vi "Top.vi"() -> ()   [LabVIEW 2020]
uses:
  PowerLineId.ctl
  PowerLineQuantity.ctl
  <vilib>/DAQmx/read.llb/DAQmx Read (Analog 1D Wfm NChan NSamp).vi
  <vilib>/DAQmx/configure/timing.llb/DAQmx Timing (Sample Clock).vi
  <vilib>/DAQmx/configure/task.llb/DAQmx Configure Logging (TDMS).vi
  <extravilib>/ChannelInstances/Messenger-a[.](wfm(dbl))/Instantiate.vi
  <extravilib>/ChannelInstances/Messenger-a[.](wfm(dbl))/Endpoint.vi
  <vilib>/DAQmx/miscellaneous.llb/DAQmx Fill In Error Info.vi
  <extravilib>/ChannelInstances/Messenger-a[.](wfm(dbl)).lvlib
panel:
  in  "Logging Mode":i32(ring)=15842 items=["Off"=10231, "Log"=15844, "Log and Read"=15842]
  in  "Data Read Interval [s]":dbl(knob)=1.0 min=1.0 max=10.0 step=1.0 scale=1.0..10.0 scale format="%#_1f"
  out "Monitor":waveform(dbl)[](graph)
  in  "STOP":bool
  in  "Rate Selection":enum32{"Auto", "Manual"}(radio)
  in  "Sampling Rate [Hz]":dbl(knob)=100000.0 min=100000.0 max=2000000.0 step=50000.0 scale=100000.0..2000000.0 scale format="%.1p"
  in  "Log File Path":path
  in  "START":bool
  in  "Channel\nIO":tag="PXIe-4309/ai2"
  in  "Channel\nPCIEVPH":tag="PXIe-4309/ai5"
  in  "Channel\nDDR_VPP":tag="PXIe-4309/ai15"
  in  "Enable Channel\nIO":bool=TRUE
  in  "Enable Channel\nPCIEVPH":bool=TRUE
  in  "Enable Channel\nDDR_VPP":bool=TRUE
  in  "Channel\nDDR_SOC":tag="PXIe-4309/ai1"
  in  "Channel\nPCIEVP":tag="PXIe-4309/ai4"
  in  "Channel\nDDR_PLL":tag="PXIe-4309/ai7"
  in  "Enable Channel\nDDR_SOC":bool=TRUE
  in  "Enable Channel\nPCIEVP":bool=TRUE
  in  "Enable Channel\nDDR_PLL":bool=TRUE
  in  "Enable Channel\nDDR_MEM":bool=TRUE
  in  "Enable Channel\nPLL":bool=TRUE
  in  "Enable Channel\nCORE":bool=TRUE
  in  "Channel\nDDR_MEM":tag="PXIe-4309/ai6"
  in  "Channel\nPLL":tag="PXIe-4309/ai3"
  in  "Channel\nCORE":tag="PXIe-4309/ai0"
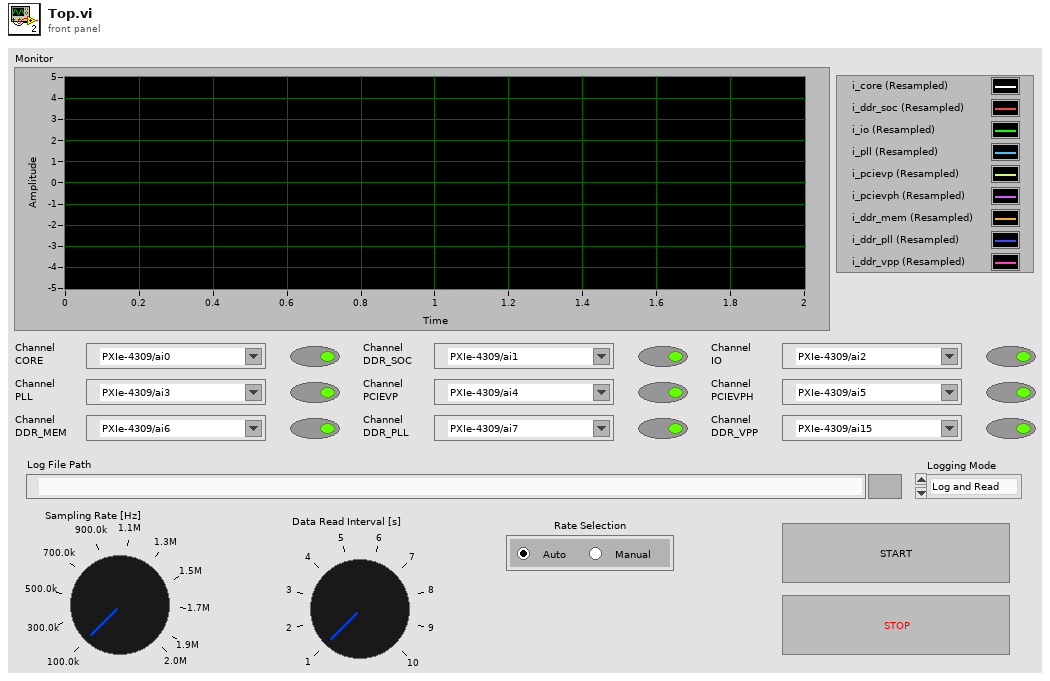
[diagram p1: front panel]
types:
  T1 = typedef "PowerLineId.ctl" = enum8{"CORE", "DDR_SOC", "IO", "PLL", "PCIEVP", "PCIEVPH", "DDR_MEM", "DDR_PLL", "DDR_VPP"}
  T2 = typedef "PowerLineQuantity.ctl" = enum16{"Current", "Voltage"}
  T3 = typedef "PowerLineConfig.ctl" = cluster{"Line Name":string, "Shunt Resistor [Ohm]":dbl, "Min Current [A]":dbl, "Max Current [A]":dbl}
  T4 = typedef "Messenger-a[.](wfm(dbl)).lvlib/))Channel.ctl" = refnum<queue>
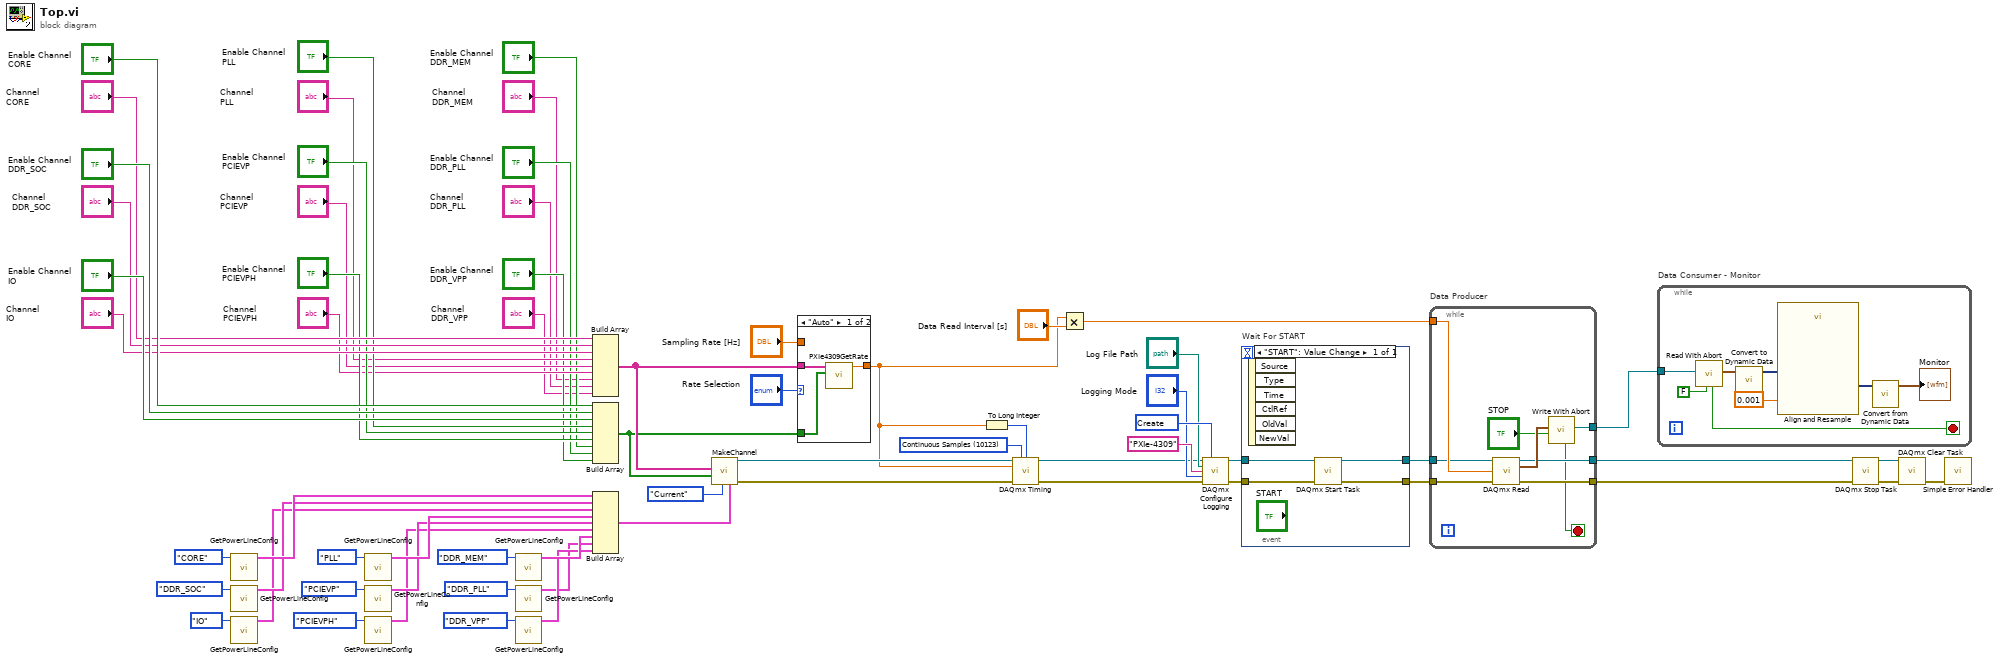
[diagram p0: block diagram]
diagram:
  w33 = 15848 items=["Open"=10437, "Open or Create"=15846, "Create or Replace"=15847, "Create"=15848] ("operation")
  w36 = 10123 items=["Finite Samples"=10178, "Continuous Samples"=10123, "Hardware Timed Single Point"=12522] ("sample mode")
  n1 = call "GetPowerLineConfig.vi"("Power Line\nIdentifier"=PowerLineId."CORE" ("Power Line Identifier")) -> ("Power Line\nConfiguration"=w64:T3)  [unwired: 8 in]
  n2 = call "GetPowerLineConfig.vi"("Power Line\nIdentifier"=PowerLineId."DDR_SOC" ("Power Line Identifier")) -> ("Power Line\nConfiguration"=w63:T3)  [unwired: 8 in]
  n3 = call "GetPowerLineConfig.vi"("Power Line\nIdentifier"=PowerLineId."IO" ("Power Line Identifier")) -> ("Power Line\nConfiguration"=w62:T3)  [unwired: 8 in]
  n4 = call "GetPowerLineConfig.vi"("Power Line\nIdentifier"=PowerLineId."PLL" ("Power Line Identifier")) -> ("Power Line\nConfiguration"=w61:T3)  [unwired: 8 in]
  n5 = call "GetPowerLineConfig.vi"("Power Line\nIdentifier"=PowerLineId."PCIEVP" ("Power Line Identifier")) -> ("Power Line\nConfiguration"=w60:T3)  [unwired: 8 in]
  n6 = call "GetPowerLineConfig.vi"("Power Line\nIdentifier"=PowerLineId."PCIEVPH" ("Power Line Identifier")) -> ("Power Line\nConfiguration"=w59:T3)  [unwired: 8 in]
  n7 = call "GetPowerLineConfig.vi"("Power Line\nIdentifier"=PowerLineId."DDR_MEM" ("Power Line Identifier")) -> ("Power Line\nConfiguration"=w58:T3)  [unwired: 8 in]
  n8 = call "GetPowerLineConfig.vi"("Power Line\nIdentifier"=PowerLineId."DDR_PLL" ("Power Line Identifier")) -> ("Power Line\nConfiguration"=w56:T3)  [unwired: 8 in]
  n9 = call "GetPowerLineConfig.vi"("Power Line\nIdentifier"=PowerLineId."DDR_VPP" ("Power Line Identifier")) -> ("Power Line\nConfiguration"=w57:T3)  [unwired: 8 in]
  n10 = Build Array("Channel\nCORE", "Channel\nDDR_SOC", "Channel\nIO", "Channel\nPLL", "Channel\nPCIEVP", "Channel\nPCIEVPH", "Channel\nDDR_MEM", "Channel\nDDR_PLL", "Channel\nDDR_VPP") -> (w27:tag[])
  n11 = Build Array("Enable Channel\nCORE", "Enable Channel\nDDR_SOC", "Enable Channel\nIO", "Enable Channel\nPLL", "Enable Channel\nPCIEVP", "Enable Channel\nPCIEVPH", "Enable Channel\nDDR_MEM", "Enable Channel\nDDR_PLL", "Enable Channel\nDDR_VPP") -> (w26:bool[])
  n12 = Build Array(w64, w63, w62, w61, w60, w59, w58, w56, w57) -> (w24:T3[])
  n13 = call "MakeChannel.vi"("Power Line\nConfigurations"=w24, "Power Line\nQuantity"=PowerLineQuantity."Current" ("Power Line\nQuantity"), "Power Line\nEnable"=w26, "Power Line\nChannels"=w27) -> ("Output Error"=w37:errorcluster, "Output Task"=w23:refnum<k21>)  [unwired: 6 in]
  n14 = case shown="\"Auto\"" "Rate Selection" {
    tunnel: w27 -> [w68 _]
    tunnel: w26 -> [w67 _]
    tunnel: [w66 w69] -> w1
    tunnel: "Sampling Rate [Hz]" -> [_ w69]
    frame "Auto" {
      n15 = call "PXIe4309GetRate.vi"("Physical Channel\nEnable"=w67, "Physical Channels"=w68) -> ("Sampling Rate"=w66:dbl)  [unwired: 9 in]
    }
    frame "Manual" {
    }
  }
  n16 = To Long Integer(number=w1) -> (32bit integer=w2:i32)
  n17 = call-poly <vilib>:"DAQmx Timing.vi"("task/channels in"=w23, "sample mode"=w36, "samples per channel"=w2, "rate"=w1, "error in"=w37) -> ("task out"=w29:refnum<k21>, "error out"=w28:errorcluster)  [unwired: 9 in]
  n18 = Multiply(x=w1, y="Data Read Interval [s]") -> (x*y=w8:dbl)
  n19 = call-poly <vilib>:"DAQmx Configure Logging.vi"("task/channels in"=w29, "operation"=w33, "file path"="Log File Path", "group name"="PXIe-4309", "logging mode"="Logging Mode", "error in"=w28) -> ("task out"=w35:refnum<k21>, "error out"=w34:errorcluster)  [unwired: 8 in]
  n20 = event "Wait For START" shown="[0] \"START\": Value Change" {
    selector: _ -> [_]
    dyn-events: _ -> [_]
    timeout: _ -> [_]
    tunnel: w35 -> [w73]
    tunnel: w34 -> [w72]
    tunnel: [w71] -> w7
    tunnel: [w70] -> w6
    event "START": Value Change {
      n21 = event-data() -> ()  [unwired: 1 in, 6 out]
      n22 = call <vilib>:"DAQmx Start Task.vi"("task/channels in"=w73, "error in"=w72) -> ("task out"=w71:refnum<k21>, "error out"=w70:errorcluster)  [unwired: 12 in]
    }
  }
  n23 = while "Data Producer" {
    tunnel: w8 -> [w81]
    tunnel: w7 -> [w80]
    tunnel: w6 -> [w79]
    tunnel: [w78] -> w5
    tunnel: [w77] -> w4
    tunnel: [w74] -> w3
    stop <- w75 stop-if-true
    n24 = call-poly <vilib>:"DAQmx Read.vi"("task/channels in"=w80, "number of samples per channel"=w81, "error in"=w79) -> ("task out"=w78:refnum<k21>, "data"=w82:waveform(dbl)[], "error out"=w77:errorcluster)  [unwired: 10 in]
    n25 = call <extravilib>:"Write With Abort.vi"("abort (F)"="STOP", "element"=w82) -> ("channel"=w74:T4, "aborted?"=w75:bool)  [unwired: 6 in, 2 out]
  }
  n26 = while "Data Consumer - Monitor" {
    tunnel: w3 -> [w90]
    stop <- w89 stop-if-true
    n27 = call <extravilib>:"Read With Abort.vi"("abort (F)"=FALSE, "channel"=w90) -> ("element"=w87:waveform(dbl)[], "aborted?"=w89:bool)  [unwired: 6 in, 2 out]
    n28 = call "Convert to Dynamic Data"("Array of Waveforms"=w87) -> ("Dynamic Data Type"=w86:dynamicdata)  [unwired: 3 in]
    n29 = call "Align and Resample"("dt"=0.001, "Signals"=w86) -> ("Resampled Signals"=w84:dynamicdata)  [unwired: 7 in, 2 out]
    n30 = call "Convert from Dynamic Data"("Dynamic Data Type"=w84) -> ("Array of Waveform"=→"Monitor":waveform(dbl)[])  [unwired: 3 in]
  }
  n31 = call <vilib>:"DAQmx Stop Task.vi"("task/channels in"=w5, "error in"=w4) -> ("task out"=w12:refnum<k21>, "error out"=w11:errorcluster)  [unwired: 12 in]
  n32 = call <vilib>:"DAQmx Clear Task.vi"("task in"=w12, "error in"=w11) -> ("error out"=w10:errorcluster)  [unwired: 13 in]
  n33 = call <vilib>:"Simple Error Handler.vi"("error in (no error)"=w10) -> ()  [unwired: 4 in, 5 out]
